vi "Auto Gyro.vi"(9 "zeroGyro":dbl, 10 "headingTarget":dbl, 11 "xSpeed":dbl) -> (3 "Finished?":bool)   [LabVIEW 2017]
uses:
  Robot Global Data.vi
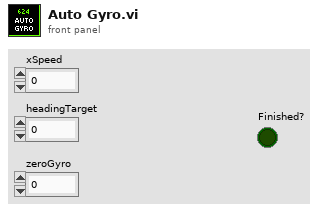
[diagram p1: front panel]
types:
  T1 = typedef "Dashboard Status Data.ctl" = cluster{"Elevator Status Cluster":T2, "Drivetrain Status Cluster":T5, "Intake Status Cluster":T8, "Climb Status Cluster":T11, "Intake PDP Info":T12}
  T2 = typedef "Elevator Status Cluster.ctl" = cluster{"Finished":bool, "Output":dbl, "Elevator State":T3, "Elevator Mode":T4, "Encoder Height":dbl, "Elevator Height":dbl, "At Bottom?":bool, "At Top?":bool}
  T3 = typedef "Elevator State.ctl" = enum16{"Idle", "Ground", "Mid", "Scale", "Switch"}
  T4 = typedef "Elevator Mode.ctl" = enum16{"Semi Auto", "Manual", "Auto"}
  T5 = typedef "Drivetrain Status Cluster.ctl" = cluster{"Throttle (Y)":dbl, "Steer (X)":dbl, "Drivetrain Mode":T6, "Brake?":bool, "Distance Drive Complete?":bool, "PID Drive Complete?":bool, "Creep Mode?":bool, "Gyro Steer Complete?":bool, "Gyro":dbl, "X Max Output":dbl, "X Min Output":dbl, "Y Max Output ":dbl, "Y Min Output":dbl, "Heading Target":dbl, "Distance Target":dbl, "Gear 2":bool, "Drivetrain Encoder Values":T7}
  T6 = typedef "Drivetrain Mode.ctl" = enum16{"Manual", "Gyro Steer", "PID Drive", "Distance Drive", "Autonomous"}
  T7 = typedef "DT Encoder Values.ctl" = cluster{"Left Encoder":cluster{"Distance":dbl, "Speed":dbl, "Tick":dbl}, "Right Encoder":cluster{"Distance":dbl, "Speed":dbl, "Tick":dbl}}
  T8 = typedef "Intake Status Cluster.ctl" = cluster{"Intake Mode":T9, "Intake States":T10, "Intake Current Angle":dbl, "Cube In Posession?":bool}
  T9 = typedef "Intake Mode.ctl" = enum16{"Auto", "Semi Auto", "Manual"}
  T10 = typedef "Intake States.ctl" = enum16{"Curl Up", "Override Angle", "Idle", "Drop Mid", "Drop Low", "Outtake", "Intake"}
  T11 = typedef "Climb Status Cluster.ctl" = cluster{"Climb":bool, "Time Remaining":dbl, "Button Pressed":bool}
  T12 = typedef "Intake PDP Info.ctl" = cluster{"Voltage Percent Output":dbl, "Output Voltage":dbl, "Bus Voltage":dbl, "Device ID":dbl, "Output Current":dbl, "Sensor Velocity":dbl, "Sensor Position":dbl, "Pulse Width Position":dbl, "Pulse Width Velocity":dbl, "Temperature":dbl, "Inverted?":bool}
  T13 = typedef "Drivetrain Command Cluster.ctl" = cluster{"Y Power":dbl, "Turn Power":dbl, "Drivetrain Mode":T6, "Gear 2":bool, "Y Min Output":dbl, "Y Max Output":dbl, "X Min Output":dbl, "X Max Output":dbl, "Heading Target":dbl, "Distance Target":dbl, "Brake?":bool, "Zero Gyro":bool}
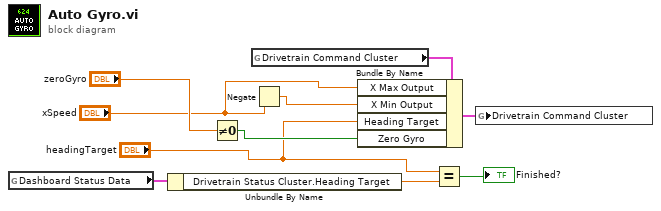
[diagram p0: block diagram]
diagram:
  n1 = global read "Robot Global Data.vi" "Dashboard Status Data"() -> (w6:T1)
  n2 = Unbundle By Name(w6) -> ("Drivetrain Status Cluster.Heading Target"=w5:dbl)
  n3 = Not Equal To 0?(x="zeroGyro") -> (x != 0?=w8:bool)
  n4 = global read "Robot Global Data.vi" "Drivetrain Command Cluster"() -> (w10:T13)
  n5 = Negate(x="xSpeed") -> (-x=w2:dbl)
  n6 = Bundle By Name(cluster=w10, "X Max Output"="xSpeed", "X Min Output"=w2, "Heading Target"="headingTarget", "Zero Gyro"=w8) -> (w9:T13)
  n7 = Equal?(x="headingTarget", y=w5) -> (x = y?=→"Finished?":bool)
  n8 = global write "Robot Global Data.vi" "Drivetrain Command Cluster"(w9) -> ()
